vi "HM8118 - Close.vi"(0 "VISA resource name":refnum<visa-resource-name>, 3 "error in (no error)":errorcluster) -> (10 "error out":errorcluster)   [LabVIEW 2017]
doc: "Performs an instrument error query before terminating the software connection to the instrument."
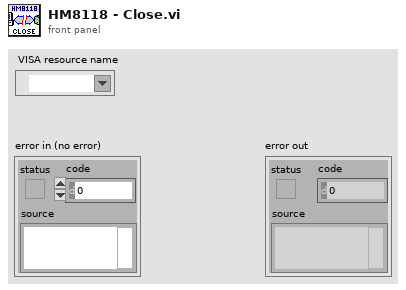
[diagram p1: front panel]
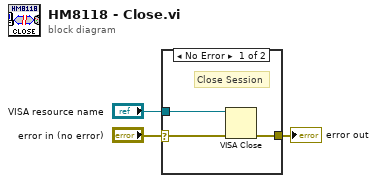
[diagram p0: block diagram]
diagram:
  n1 = case shown="No Error" "error in (no error)" {
    selector: "error in (no error)" -> [w4 w7]
    tunnel: [w6 w7] -> w3
    tunnel: "VISA resource name" -> [w5 _]
    frame No Error {
      # "Close Session"
      n2 = VISA Close(VISA resource name=w5, error in (no error)=w4) -> (error out=w6:errorcluster)
    }
    frame Error {
    }
  }
  "error out" <- w3
